vi "Register and Unregister Feeds.vi"() -> ()   [LabVIEW 2014]
doc: "This example shows how to register a feed, unregister a feed, and list all the registered feeds on the current system."
uses:
  _support/feed.ctl
  NIPM_API.lvlib
panel:
  in  "Feed name (unregister)":string caption="Feed name"
  in  "Unregister feed?":bool
  in  "Feed URI":string
  in  "Feed name (register)":string caption="Feed name"
  in  "Register feed?":bool
  out "Registered feeds on this system":T1[](array[typedef])
  # "1. In the Register Feed section, set the Register feed control to TRUE if you want to register a feed.  Then specify the Feed name and Feed URI\n2. In the Unregister Feed section, set the Unregister feed control to TRUE if you want to unregister a feed.  Then specify the Feed name.\n3. Run the VI."
  # "Register Feed"
  # "Unregister Feed"
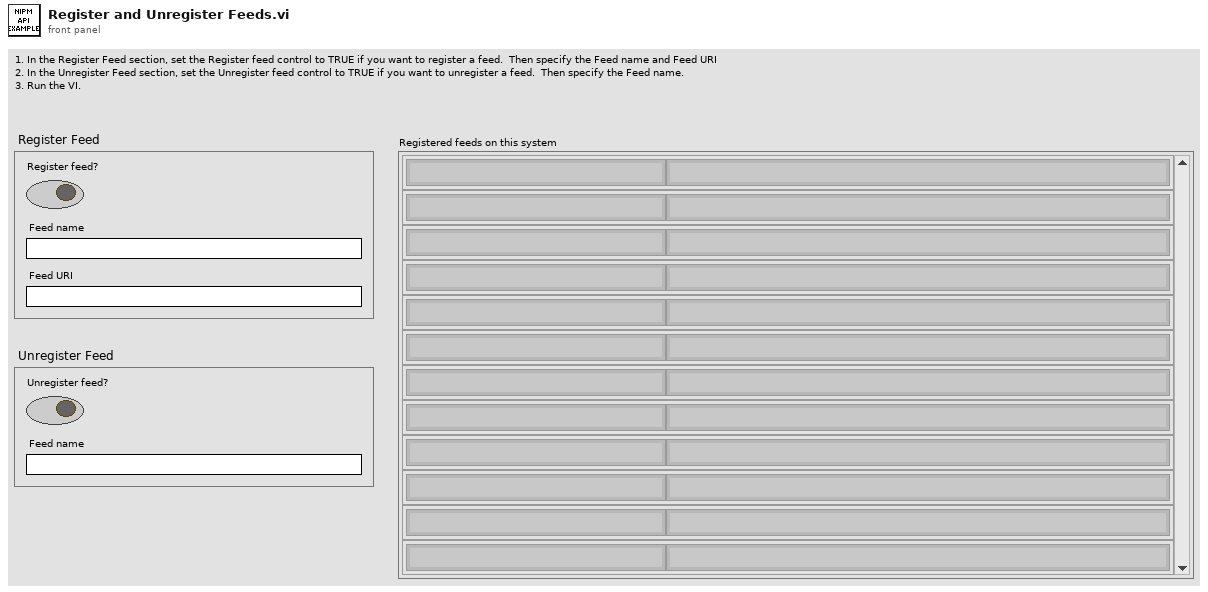
[diagram p1: front panel]
types:
  T1 = typedef "NIPM_API.lvlib/feed.ctl" = cluster{"Name":string, "URI":string}
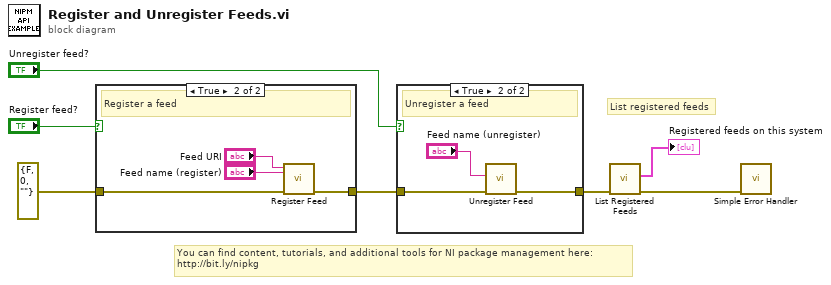
[diagram p0: block diagram]
diagram:
  # "List registered feeds"
  # "You can find content, tutorials, and additional tools for NI package management here:\nhttp://bit.ly/nipkg"
  n1 = case shown="True" "Register feed?" {
    tunnel: [w8 w10] -> w3
    tunnel: errorcluster {"status"=FALSE, "code"=0, "source"=""} ("error in") -> [w8 w9]
    frame False {
      # "Do nothing"
    }
    frame True {
      # "Register a feed"
      n2 = call "Register Feed.vi"("error in"=w9, "feed name"="Feed name (register)", "feed URI"="Feed URI") -> ("error out"=w10:errorcluster)  [unwired: 7 in, 1 out]
    }
  }
  n3 = case shown="True" "Unregister feed?" {
    tunnel: [w13 w16] -> w2
    tunnel: w3 -> [w13 w15]
    frame False {
      # "Do nothing"
    }
    frame True {
      # "Unregister a feed"
      n4 = call "Unregister Feed.vi"("error in"=w15, "feed name"="Feed name (unregister)") -> ("error out"=w16:errorcluster)  [unwired: 8 in, 1 out]
    }
  }
  n5 = call "List Registered Feeds.vi"("error in"=w2) -> ("error out"=w1:errorcluster, "registered feeds"=→"Registered feeds on this system":T1[])  [unwired: 9 in]
  n6 = call <vilib>:"Simple Error Handler.vi"("error in (no error)"=w1) -> ()  [unwired: 4 in, 5 out]
